vi "_CSMObj-Append Chain Node.vi"(7 "Allowed Messages(Empty for all)":string[](array[string]), 8 "Error in":errorcluster caption="Error in (no error)", 10 "Requested Name":string, 11 "CSMObj in":T1={"Requested Name"="", "Module Name"="", "Mode"=enum."Stand Alone", "Queue"=refnum, "CSM-Data"=refnum, "User Event"=refnum, "Status Change Event"=refnum, "Allowed Messages"=[], "Mode-Data"=refnum, "Group Name"="", "Exit Event"=refnum}) -> (0 "Error out":errorcluster, 2 "output cluster (dup)":T1={"Requested Name"="", "Module Name"="", "Mode"=enum."Stand Alone", "Queue"=refnum, "CSM-Data"=refnum, "User Event"=refnum, "Status Change Event"=refnum, "Allowed Messages"=[], "Mode-Data"=refnum, "Group Name"="", "Exit Event"=refnum}, 3 "CSMObj out":T1={"Requested Name"="", "Module Name"="", "Mode"=enum."Stand Alone", "Queue"=refnum, "CSM-Data"=refnum, "User Event"=refnum, "Status Change Event"=refnum, "Allowed Messages"=[], "Mode-Data"=refnum, "Group Name"="", "Exit Event"=refnum})   [LabVIEW 2020, in "Communicable State Machine.lvlib"]
uses:
  Communicable State Machine.lvlib
  _CSMObj.ctl
  Priority Queue.lvclass
  _CSM_MODE.ctl
  _CSMObj-Data.ctl
  _CSM Status Change Event Data.ctl
  _CSMObj-ModeData.ctl
  Priority Queue.lvclass/Priority Queue.ctl
  Obtain Priority Queue.vi
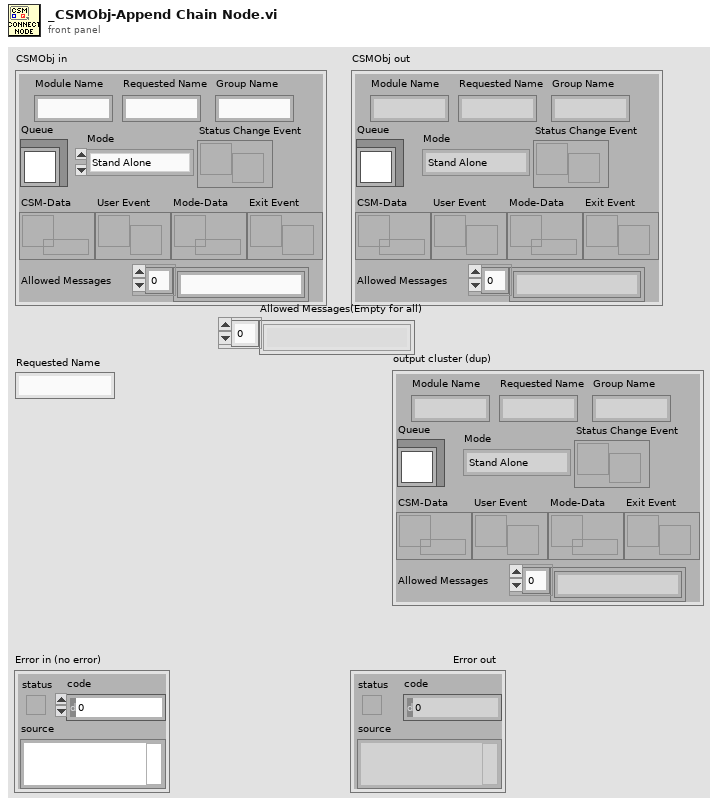
[diagram p1: front panel]
types:
  T1 = typedef "Communicable State Machine.lvlib/_CSMObj.ctl" = cluster{"Requested Name":string, "Module Name":string, "Mode":T2, "Queue":refnum<class "Priority Queue.lvclass">, "CSM-Data":refnum<data-value>, "User Event":refnum<user-event>, "Status Change Event":refnum<user-event>, "Allowed Messages":string[], "Mode-Data":refnum<data-value>, "Group Name":string, "Exit Event":refnum<user-event>}
  T2 = typedef "Communicable State Machine.lvlib/_CSM_MODE.ctl" = enum16{"Not Exist", "Stand Alone", "CSM", "Worker Agent", "Worker", "Chain", "Chain Node"}
  T3 = typedef "Communicable State Machine.lvlib/_CSMObj-Data.ctl" = cluster{"RemoteMessge?":bool, "error":errorcluster}
  T4 = typedef "Communicable State Machine.lvlib/_CSM_NAME_REQUEST.ctl" = enum16{"Stand Alone CSM Request", "Normal CSM Request", "Agent Request", "Action Worker Request", "Chain Request", "Chain Node Request"}
  T5 = typedef "Communicable State Machine.lvlib/_CSM Status Change Event Data.ctl" = cluster{"ModuleName":string, "Status":string, "Arguments":string}
  T6 = cluster{"Requested Name":string, "Allowed Messages(Empty for all)":string[]}
  T7 = typedef "Communicable State Machine.lvlib/_CSMObj-ModeData.ctl" = cluster{"Share Count":i32, "Messages of Chain Nodes":cluster{"Module Name":string, "Allowed Messages":string[]}[], "Chain Message Mapping Map":variant}
  T8 = cluster{"Module Name":string, "Allowed Messages":string[]}[]
  T9 = cluster{"Requested Name":string, "Allowed Messages(Empty for all)":string[]}[]
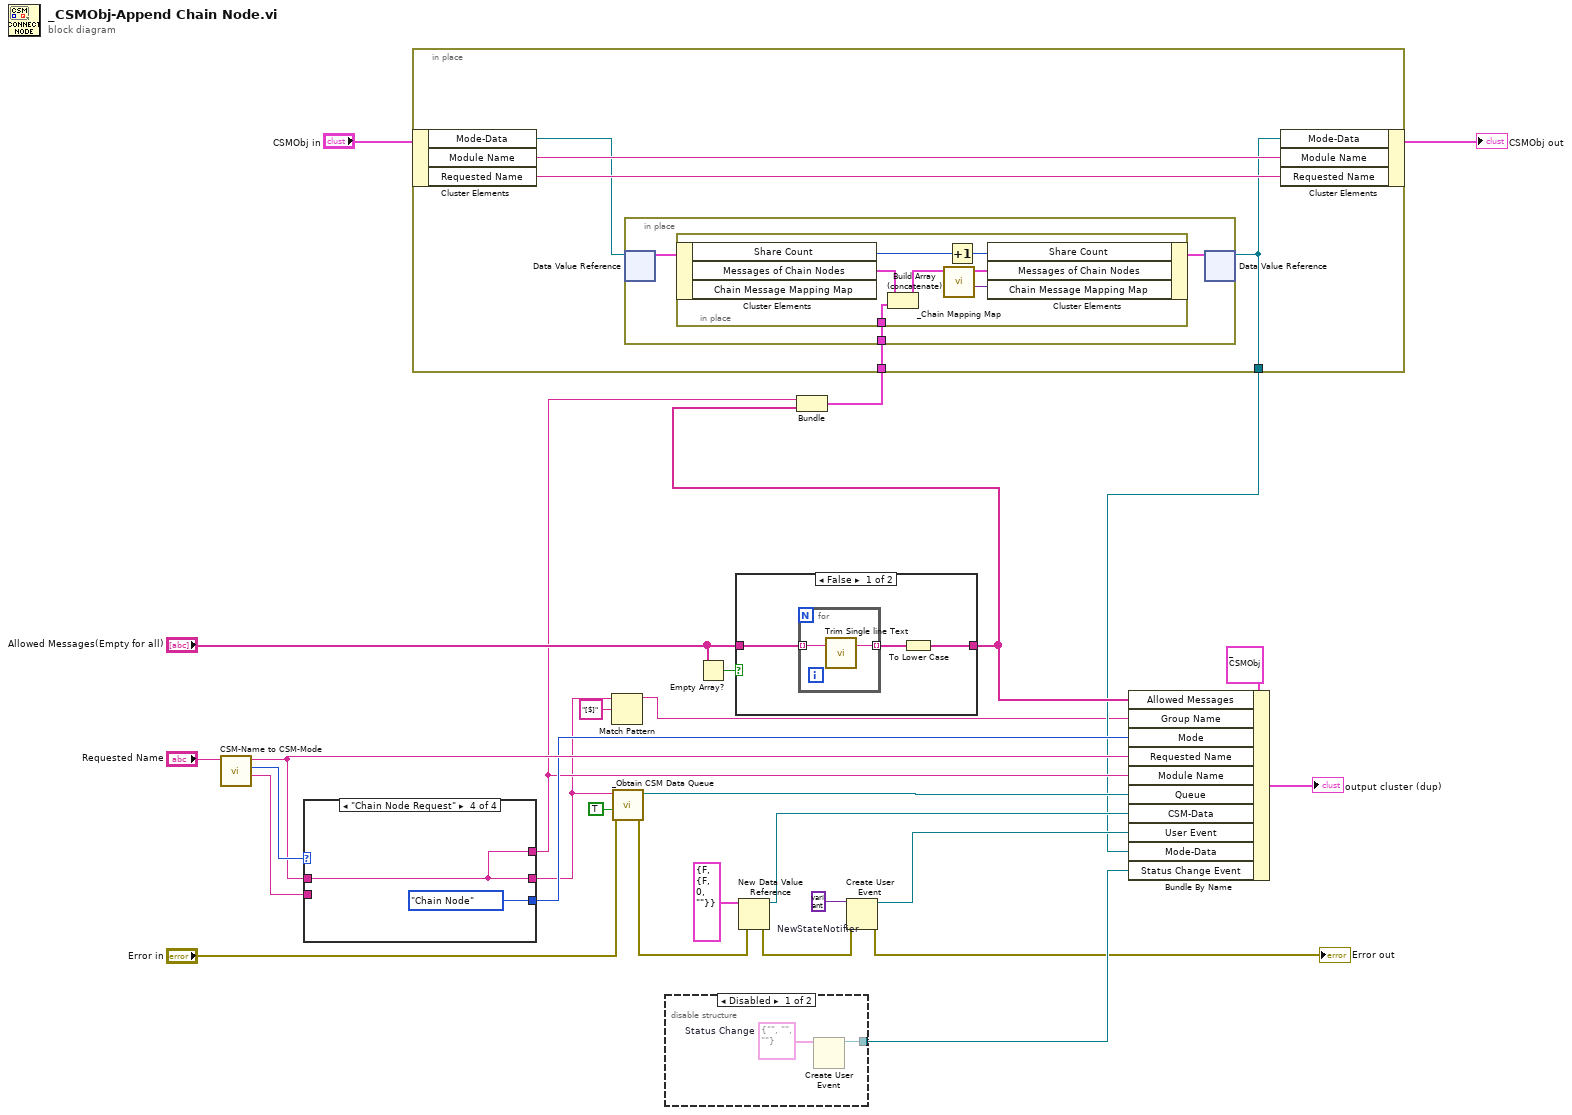
[diagram p0: block diagram]
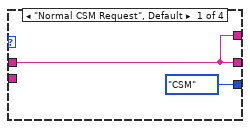
[diagram p2: hidden frame]
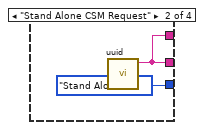
[diagram p3: hidden frame]
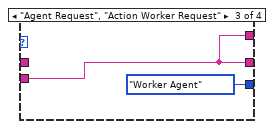
[diagram p4: hidden frame]
diagram:
  w23 = variant  # NewStateNotifier
  n1 = call "CSM-Name to CSM-Mode.vi"("String"="Requested Name") -> ("ParentCSM Name"=w16:string, "CSM Mode"=w15:T4, "Requested Name"=w14:string)  [unwired: 8 in]
  n2 = case shown="\"Chain Node Request\"" w15 {
    tunnel: [w30 w32 w34 w36] -> w3
    tunnel: w14 -> [w30 _ _ w36]
    tunnel: w16 -> [_ _ w34 _]
    tunnel: [_CSM_MODE."CSM" ("Mode") _CSM_MODE."Stand Alone" ("Mode") _CSM_MODE."Worker Agent" ("Mode") _CSM_MODE."Chain Node" ("Mode")] -> w13
    tunnel: [w30 w32 w34 w36] -> w6
    frame "Normal CSM Request", Default {
    }
    frame "Stand Alone CSM Request" {
      n3 = call "uuid.vi"() -> ("UUID"=w32:string)  [unwired: 11 in]
    }
    frame "Agent Request", "Action Worker Request" {
    }
    frame "Chain Node Request" {
    }
  }
  n4 = Match Pattern(string=w3, regular expression="[$]") -> (before substring=w1:string)  [unwired: 1 in, 3 out]
  n5 = call "_Obtain CSM Data Queue.vi"("error in (no error)"="Error in", "create if not found? (T)"=TRUE, "Name"=w3) -> ("error out"=w24:errorcluster, "Priority Queue"=w26:refnum<class "Priority Queue.lvclass">)  [unwired: 6 in, 1 out]
  n6 = disable-structure shown="Disabled" {
    disable-tunnel: [w38 _] -> w20
    frame Disabled {
      w39 = T5 {"ModuleName"="", "Status"="", "Arguments"=""}  # Status Change
      n7 = Create User Event(user event datatype=w39) -> (user event=w38:refnum<user-event>)  [unwired: 1 in, 1 out]
    }
    frame Enabled {
    }
  }
  n8 = Empty Array?(array="Allowed Messages(Empty for all)") -> (empty?=w17:bool)
  n9 = case shown="False" w17 {
    tunnel: [w40 w45] -> w5
    tunnel: "Allowed Messages(Empty for all)" -> [w41 w45]
    frame False {
      n10 = for {
        tunnel: [w43] -> w42 mode=indexing
        tunnel: w41 -> [w44] mode=indexing
        n11 = call "Trim Single line Text.vi"("single-line text"=w44) -> ("trimed text"=w43:string)  [unwired: 2 in]
      }
      n12 = To Lower Case(string=w42) -> (all lower case string=w40:string[])
    }
    frame True {
    }
  }
  n13 = New Data Value Reference(data value=T3 {"RemoteMessge?"=FALSE, "error"={"status"=FALSE, "code"=0, "source"=""}} ("CSMObj-Data"), error in=w24) -> (data value reference=w25:refnum<data-value>, error out=w22:errorcluster)
  n14 = Bundle("Requested Name"=w6, "Allowed Messages(Empty for all)"=w5) -> (w27:T6)  [unwired: 1 in]
  n15 = in-place "In Place Element Structure" {
    in-place-border: w27 -> [w47]
    in-place-border: [w46] -> w4
    n16 = in-place-cluster #1("CSMObj in") -> ("Mode-Data"=w48:refnum<data-value>, "Module Name"=w50:string, "Requested Name"=w49:string)
    n17 = in-place {
      in-place-border: w47 -> [w51]
      n18 = in-place-dvr #2(w48) -> (w53:T7)  [unwired: 1 out]
      n19 = in-place {
        in-place-border: w51 -> [w57]
        n20 = in-place-cluster #3(w53) -> ("Share Count"=w60:i32, "Messages of Chain Nodes"=w58:T8)  [unwired: 1 out]
        n21 = Build Array (concatenate)(w58, w57) -> (w56:T9)
        n22 = call "_Chain Mapping Map.vi"("Messages of Chain Nodes"=w56) -> ("variant"=w54:variant, "Messages of Chain Nodes (dup)"=w55:T8)  [unwired: 9 in]
        n23 = Increment(x=w60) -> (x+1=w59:i32)
        n24 = in-place-cluster #3("Share Count"=w59, "Messages of Chain Nodes"=w55, "Chain Message Mapping Map"=w54) -> (w52:T7)
      }
      n25 = in-place-dvr #2(w52) -> (w46:refnum<data-value>)  [unwired: 1 out]
    }
    n26 = in-place-cluster #1("Mode-Data"=w46, "Module Name"=w50, "Requested Name"=w49) -> (→"CSMObj out":T1)
  }
  n27 = Create User Event(user event datatype=w23, error in=w22) -> (user event=w21:refnum<user-event>, error out=→"Error out":errorcluster)
  n28 = Bundle By Name(cluster=T1 {"Requested Name"="", "Module Name"="", "Mode"=enum."Stand Alone", "Queue"=refnum, "CSM-Data"=refnum, "User Event"=refnum, "Status Change Event"=refnum, "Allowed Messages"=[], "Mode-Data"=refnum, "Group Name"="", "Exit Event"=refnum} ("CSMQ in"), "Allowed Messages"=w5, "Group Name"=w1, "Mode"=w13, "Requested Name"=w14, "Module Name"=w6, "Queue"=w26, "CSM-Data"=w25, "User Event"=w21, "Mode-Data"=w4, "Status Change Event"=w20) -> (→"output cluster (dup)":T1)
